vi "MotionStop.vi"(8 "error in (no error)":errorcluster, 11 "Tapedrive_ESP301 in":refnum<class "Tapedrive_ESP301.lvclass">) -> (0 "error out":errorcluster, 2 "new command":string, 3 "Tapedrive_ESP301 out":refnum<class "Tapedrive_ESP301.lvclass">)   [LabVIEW 2011, in "Tapedrive_ESP301.lvclass"]
uses:
  Tapedrive_ESP301.lvclass
  Tapedrive_ESP301.lvclass/Tapedrive_ESP301.ctl
  Newport ESP301.lvlib
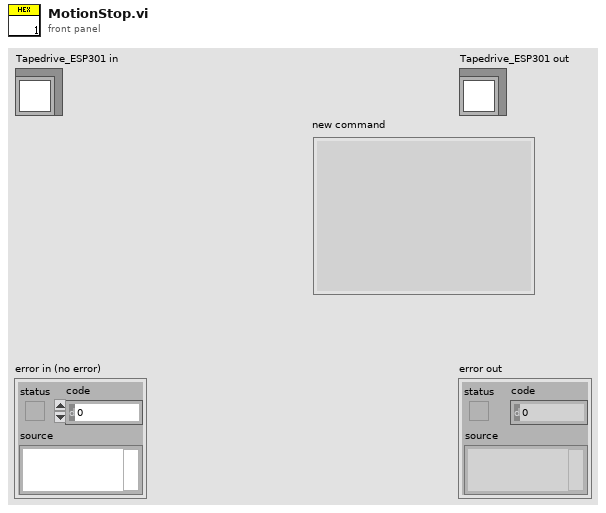
[diagram p1: front panel]
types:
  T1 = typedef "OnOffTypeDef.ctl" = enum16{"off", "on"}
  T2 = typedef "Direction.ctl" = enum16{"Forward", "Backward", "Undefined"}
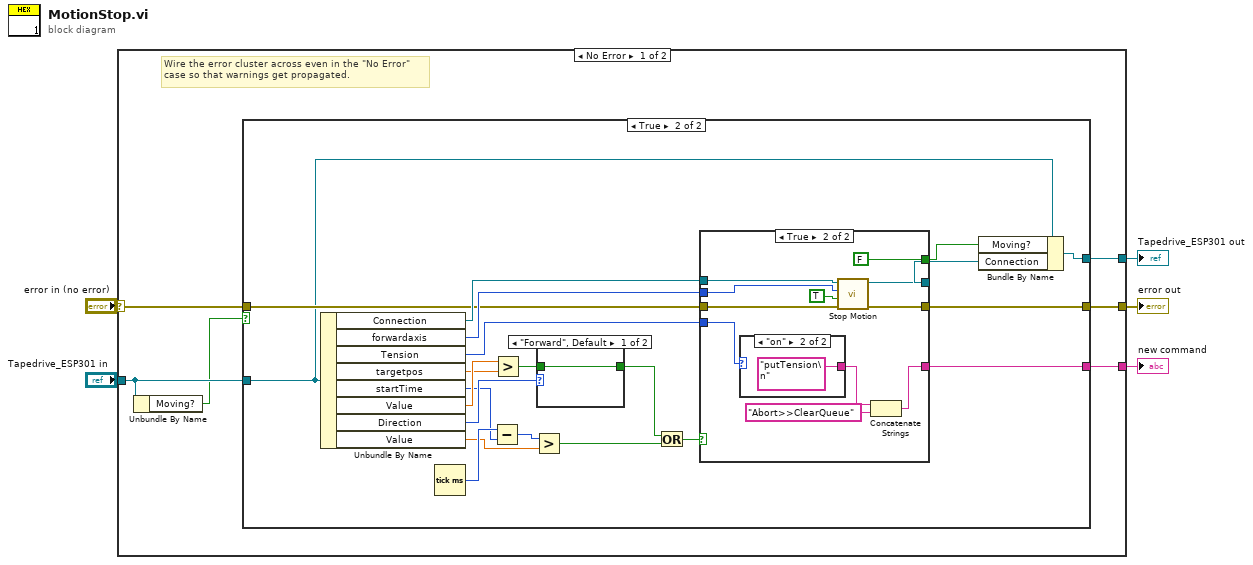
[diagram p0: block diagram]
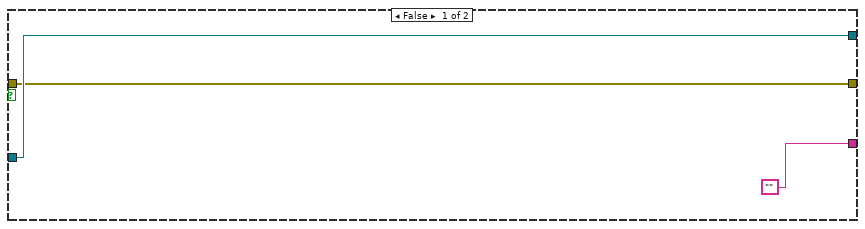
[diagram p2: hidden frame]
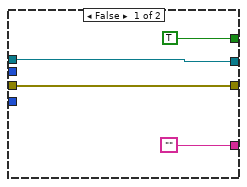
[diagram p3: hidden frame]
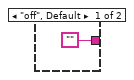
[diagram p4: hidden frame]
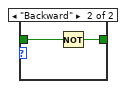
[diagram p5: hidden frame]
diagram:
  n1 = case shown="No Error" "error in (no error)" {
    selector: "error in (no error)" -> [w9 w57]
    tunnel: [w10 w57] -> w4
    tunnel: [w11 w56] -> w2
    tunnel: "Tapedrive_ESP301 in" -> [w7 w56]
    tunnel: [w8 _] -> w1
    frame No Error {
      # "Wire the error cluster across even in the \"No Error\"\ncase so that warnings get propagated."
      n2 = Unbundle By Name(w7) -> ("Moving?"=w6:bool)
      n3 = case shown="True" w6 {
        tunnel: [w14 w21] -> w11
        tunnel: [w13 w19] -> w10
        tunnel: w9 -> [w13 w18]
        tunnel: ["" w17] -> w8
        tunnel: w7 -> [w14 w15]
        frame False {
        }
        frame True {
          n4 = Unbundle By Name(w15) -> ("Connection"=w22:refnum<visa-resource-name>, "forwardaxis"=w23:i16, "Tension"=w24:T1, "targetpos"=w34:dbl, "startTime"=w30:u32, "Value"=w35:dbl, "Direction"=w33:T2, "Value"=w28:dbl)
          n5 = Tick Count (ms)() -> (millisecond timer value=w31:u32)
          n6 = Subtract(x=w31, y=w30) -> (x-y=w29:u32)
          n7 = Greater?(x=w35, y=w34) -> (0:w32:bool)
          n8 = Greater?(x=w29, y=w28) -> (0:w27:bool)
          n9 = case shown="\"Forward\", Default" w33 {
            tunnel: [w53 w54] -> w26
            tunnel: w32 -> [w53 w55]
            frame "Forward", Default {
            }
            frame "Backward" {
              n10 = Not(x=w55) -> (.not. x?=w54:bool)
            }
          }
          n11 = Or(x=w26, y=w27) -> (x .or. y?=w25:bool)
          n12 = case shown="True" w25 {
            tunnel: w24 -> [_ w50]
            tunnel: w23 -> [_ w49]
            tunnel: w22 -> [w39 w48]
            tunnel: w18 -> [w38 w47]
            tunnel: [w38 w43] -> w19
            tunnel: [w39 w44] -> w16
            tunnel: ["" w40] -> w17
            tunnel: [TRUE ("Wait for Step") FALSE ("Wait for Step")] -> w20
            frame False {
            }
            frame True {
              n13 = case shown="\"on\"" w50 {
                tunnel: ["" "putTension\n"] -> w42
                frame "off", Default {
                }
                frame "on" {
                }
              }
              n14 = call "Stop Motion.vi"("error in (no error)"=w47, "Stop all axes (F)"=TRUE, "Axis (1)"=w49, "VISA resource name"=w48) -> ("error out"=w43:errorcluster, "VISA resource name out"=w44:refnum<visa-resource-name>)  [unwired: 2 in]
              n15 = Concatenate Strings(w42, "Abort>>ClearQueue" ("string")) -> (w40:string)
            }
          }
          n16 = Bundle By Name(cluster=w15, "Moving?"=w20, "Connection"=w16) -> (w21:refnum<class "Tapedrive_ESP301.lvclass">)
        }
      }
    }
    frame Error {
    }
  }
  "error out" <- w4
  "Tapedrive_ESP301 out" <- w2
  "new command" <- w1
